vi "Read General File.vi"(8 "error in (no error)":errorcluster, 10 "Session":string, 11 "path":path) -> (0 "error out":errorcluster, 1 "Controle":string, 2 "Padrao":string, 3 "path":path, 4 "Patrim":string, 5 "Data":string, 6 "Hoje":string)   [LabVIEW 2015]
uses:
  <vilib>/Utility/config.llb/Read Key (Path).vi
  <vilib>/Utility/config.llb/Read Key (String).vi
  <vilib>/Utility/config.llb/NI_LVConfig.lvlib
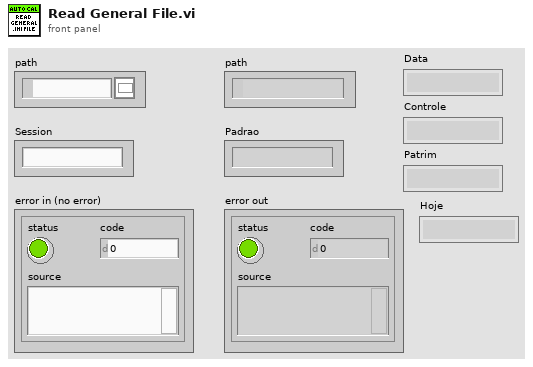
[diagram p1: front panel]
types:
  T1 = typedef "NI_LVConfig.lvlib/Config Data RefNum.ctl" = refnum<k1>
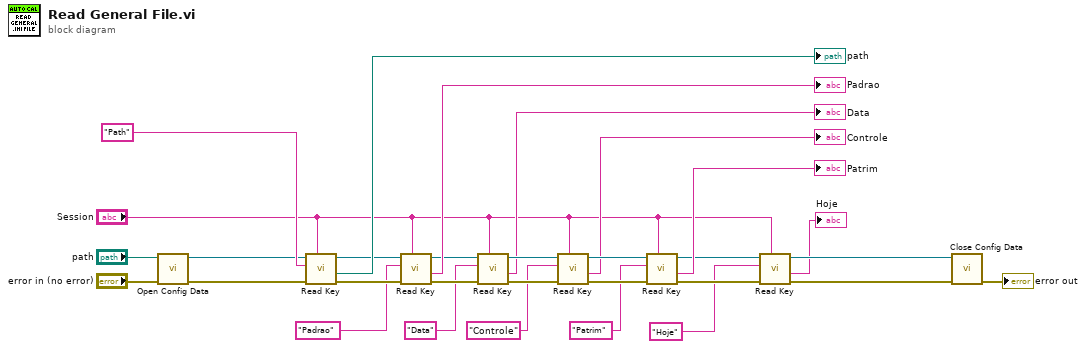
[diagram p0: block diagram]
diagram:
  n1 = call <vilib>:"Open Config Data.vi"("error in (no error)"="error in (no error)", "configuration file path"="path") -> ("error out"=w9:errorcluster, "refnum"=w8:T1)  [unwired: 7 in, 1 out]
  n2 = call-poly <vilib>:"Read Key.vi"("section"="Session", "error in (no error)"=w9, "key"="Path", "refnum"=w8) -> ("error out"=w29:errorcluster, "value"=→"path":path, "refnum out"=w25:T1)  [unwired: 4 in, 1 out]
  n3 = call-poly <vilib>:"Read Key.vi"("section"="Session", "error in (no error)"=w29, "key"="Padrao", "refnum"=w25) -> ("error out"=w16:errorcluster, "value"=→"Padrao":string, "refnum out"=w21:T1)  [unwired: 4 in, 1 out]
  n4 = call-poly <vilib>:"Read Key.vi"("section"="Session", "error in (no error)"=w16, "key"="Data", "refnum"=w21) -> ("error out"=w17:errorcluster, "value"=→"Data":string, "refnum out"=w20:T1)  [unwired: 4 in, 1 out]
  n5 = call-poly <vilib>:"Read Key.vi"("section"="Session", "error in (no error)"=w17, "key"="Controle", "refnum"=w20) -> ("error out"=w18:errorcluster, "value"=→"Controle":string, "refnum out"=w19:T1)  [unwired: 4 in, 1 out]
  n6 = call-poly <vilib>:"Read Key.vi"("section"="Session", "error in (no error)"=w18, "key"="Patrim", "refnum"=w19) -> ("error out"=w6:errorcluster, "value"=→"Patrim":string, "refnum out"=w7:T1)  [unwired: 4 in, 1 out]
  n7 = call-poly <vilib>:"Read Key.vi"("section"="Session", "error in (no error)"=w6, "key"="Hoje", "refnum"=w7) -> ("error out"=w5:errorcluster, "value"=→"Hoje":string, "refnum out"=w4:T1)  [unwired: 4 in, 1 out]
  n8 = call <vilib>:"Close Config Data.vi"("error in (no error)"=w5, "refnum"=w4) -> ("error out"=→"error out":errorcluster)  [unwired: 8 in, 1 out]
